vi "ACNET Device Checker via RPC.vi"(1 "Device":string="d:outtmp") -> (0 "Value":dbl)   [LabVIEW 2013]
uses:
  <vilib>/Utility/error.llb/DialogType.ctl
panel:
  in  "Data in 2":string="</string></value>\n</param>\n</params>\n</methodCall>\n\""
  out "after substring":string
  in  "address":string="www-bd.fnal.gov"
  out "data out":string
  in  "Data in":string="POST /xmlrpc/Accelerator HTTP/1.0\r\nContent-Type: text/xml\r\nContent-Length: 161\r\n\r\n<?xml version='1.0'?>\n<methodCall>\n<methodName>getReading</methodName>\n<params>\n<param>\n<value><string>"
  # "by Dave Peterson\nUpdated 11/11/05"
  # "www-bd.fnal.gov"
  # "131.225.121.145"
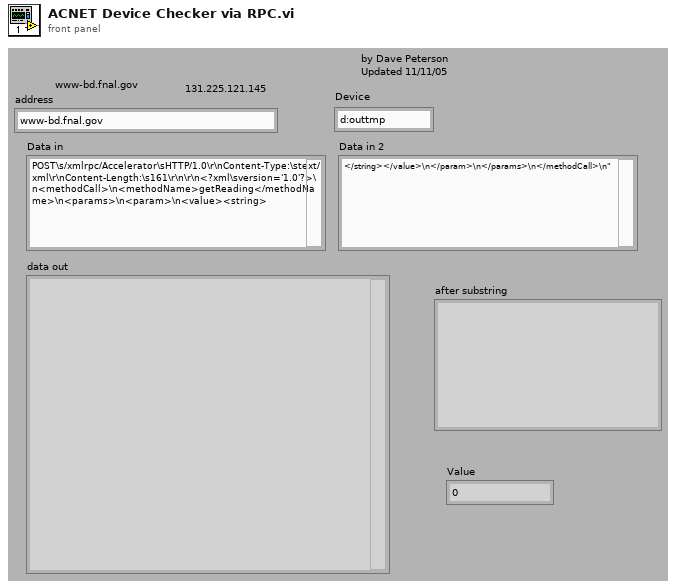
[diagram p1: front panel]
types:
  T1 = typedef "DialogType.ctl" = u16
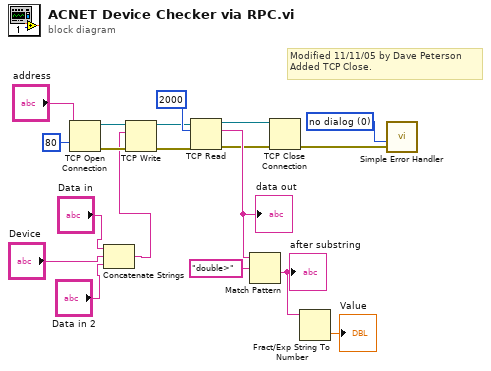
[diagram p0: block diagram]
diagram:
  w14 = T1 0 items=["no dialog", "OK message", "continue or stop message", "OK message + warnings", "continue/stop + warnings"] ("type of dialog (OK msg:1)")
  # "Modified 11/11/05 by Dave Peterson\nAdded TCP Close."
  n1 = TCP Open Connection(address="address", remote port or service name=u16 80 ("remote port")) -> (connection ID=w18:refnum<k5>, error out=w17:errorcluster)  [unwired: 3 in]
  n2 = Concatenate Strings("Data in", "Device", "Data in 2") -> (w6:string)
  n3 = TCP Write(connection ID=w18, data in=w6, error in (no error)=w17) -> (connection ID out=w13:refnum<k5>, error out=w12:errorcluster)  [unwired: 1 in, 1 out]
  n4 = TCP Read(connection ID=w13, bytes to read=2000, error in (no error)=w12) -> (connection ID out=w1:refnum<k5>, data out=w11:string, error out=w3:errorcluster)  [unwired: 2 in]
  "data out" <- w11
  n5 = Match Pattern(string=w11, regular expression="double>") -> (after substring=w9:string)  [unwired: 1 in, 3 out]
  "after substring" <- w9
  n6 = TCP Close Connection(connection ID=w1, error in (no error)=w3) -> (error out=w2:errorcluster)  [unwired: 1 in, 1 out]
  n7 = Fract/Exp String To Number(string=w9) -> (number=→"Value":dbl)  [unwired: 3 in, 1 out]
  n8 = call <vilib>:"Simple Error Handler.vi"("type of dialog (OK msg:1)"=w14, "error in (no error)"=w2) -> ()  [unwired: 3 in, 5 out]
